vi "StopClone.vi"(8 "error in (no error)":errorcluster, 9 "Wait for Module to stop?":bool, 11 "ModuleAdmin":refnum<class "ModuleAdmin.lvclass">) -> (0 "error out":errorcluster)   [LabVIEW 2014, in "NetworkImpairmentModule.lvlib"]
uses:
  NetworkImpairmentModule.lvlib
  <userlib>/NIST/ModuleAdminLib/ModuleAdmin/ModuleAdmin.lvclass
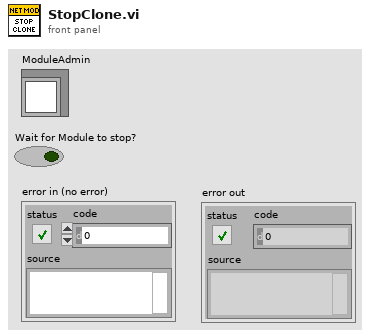
[diagram p1: front panel]
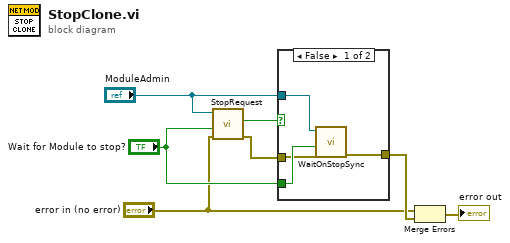
[diagram p0: block diagram]
diagram:
  n1 = call "StopRequest.vi"("error in (no error)"="error in (no error)", "Wait for Module to stop? (F)"="Wait for Module to stop?", "ModuleAdmin"="ModuleAdmin") -> ("error out"=w2:errorcluster, "Stop Request Sent"=w3:bool)  [unwired: 7 in]
  n2 = case shown="False" w3 {
    tunnel: "Wait for Module to stop?" -> [w11 _]
    tunnel: [w10 w12] -> w6
    tunnel: w2 -> [w9 w12]
    tunnel: "ModuleAdmin" -> [w8 _]
    frame False {
      n3 = call <userlib>:"WaitOnStopSync.vi"("error in (no error)"=w9, "WaitForModuleToStop?"=w11, "ModuleAdmin"=w8) -> ("error out"=w10:errorcluster)  [unwired: 7 in, 1 out]
    }
    frame True {
    }
  }
  n4 = Merge Errors("error in (no error)", w6) -> (→"error out":errorcluster)
